vi "GraphCurve.vi"(8 "error in (no error)":errorcluster caption="entrée d'erreur (pas d'erreur)", 9 "CurvIndex":i32, 10 "Curve Name":string, 11 "Interface en entrée":refnum<class "Interface.lvclass"> caption="DNL_LabVIEW Object in") -> (0 "error out":errorcluster caption="sortie d'erreur", 3 "Interface en sortie":refnum<class "Interface.lvclass"> caption="DNL_LabVIEW Object out")   [LabVIEW 2019, in "Interface.lvclass"]
uses:
  Interface.lvclass
  Interface.lvclass/Interface.ctl
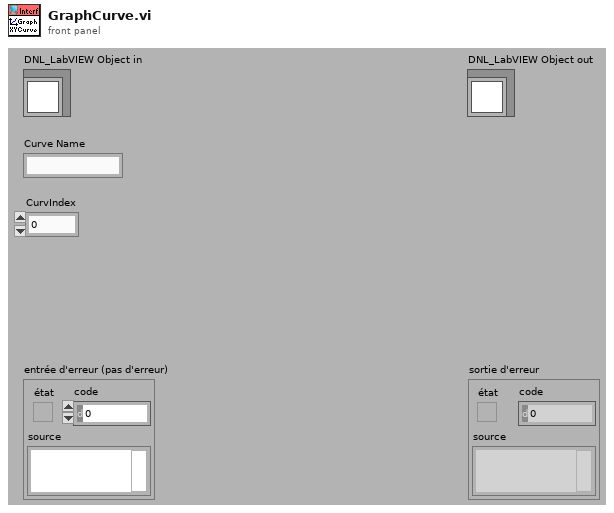
[diagram p1: front panel]
types:
  T1 = typedef "Interface.lvclass/CurveSetup.ctl" = cluster{"CurveName":string, "YParam":string, "XParam":string, "ZParam ":string, "GroupName":string, "LinWdth":u8, "PntCol":u32, "LinCol":u32, "LablFor":u8, "XScale":u32, "YScale":u32, "Interpol":u8, "DisplayName":string, "FillType":i16, "LineStyle":u8, "PntStyle":u8, "BarTyp":u8, "GraphIndex":i32, "Visible":bool, "XScaleName":string, "YScaleName":string, "XYGraph_Ref":refnum<vi>, "Data Only":bool, "DataQ Ref":refnum<queue>, "XParQ Ref":refnum<queue>, "XParamInd":i32, "ScanInd":i32, "File Path":path}
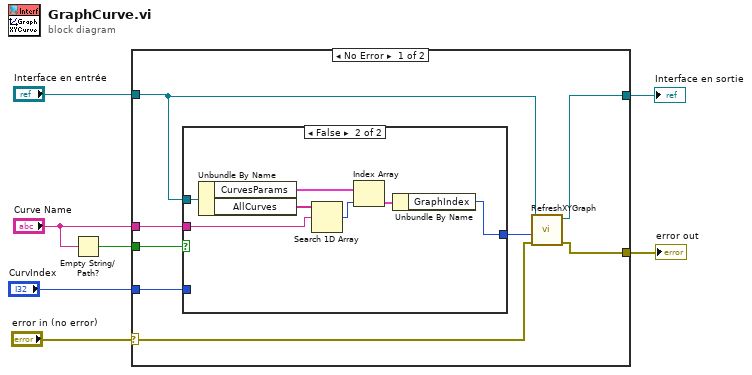
[diagram p0: block diagram]
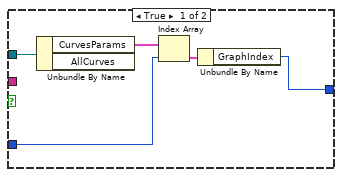
[diagram p2: hidden frame]
diagram:
  n1 = Empty String/Path?(string/path="Curve Name") -> (empty?=w2:bool)
  n2 = case shown="No Error" "error in (no error)" {
    selector: "error in (no error)" -> [w14 w29]
    tunnel: [w11 w29] -> w6
    tunnel: [w12 w28] -> w4
    tunnel: "Interface en entrée" -> [w13 w28]
    tunnel: "Curve Name" -> [w15 _]
    tunnel: w2 -> [w10 _]
    tunnel: "CurvIndex" -> [w9 _]
    frame No Error {
      n3 = case shown="False" w10 {
        tunnel: w15 -> [_ w26]
        tunnel: [w17 w21] -> w8
        tunnel: w13 -> [w20 w25]
        tunnel: w9 -> [w16 _]
        frame True {
          n4 = Unbundle By Name(w20) -> ("CurvesParams"=w19:T1[])  [unwired: 1 out]
          n5 = Index Array(array=w19, index=w16) -> (element=w18:T1)
          n6 = Unbundle By Name(w18) -> ("GraphIndex"=w17:i32)
        }
        frame False {
          n7 = Unbundle By Name(w25) -> ("CurvesParams"=w24:T1[], "AllCurves"=w27:string[])
          n8 = Search 1D Array(1D array=w27, element=w26) -> (index of element=w23:i32)  [unwired: 1 in]
          n9 = Index Array(array=w24, index=w23) -> (element=w22:T1)
          n10 = Unbundle By Name(w22) -> ("GraphIndex"=w21:i32)
        }
      }
      n11 = call "RefreshXYGraph.vi"("error in (no error)"=w14, "Graph Index"=w8, "Interface en entrée"=w13) -> ("error out"=w11:errorcluster, "Interface en sortie"=w12:refnum<class "Interface.lvclass">)  [unwired: 6 in, 1 out]
    }
    frame Error {
    }
  }
  "error out" <- w6
  "Interface en sortie" <- w4
